vi "MGCC_FntStaMach_Visitualization.vi"() -> ()   [LabVIEW 2016]
uses:
  <vilib>/DNP3/DNP3_Master/Response Type.ctl
  <vilib>/DNP3/DNP3_Master.lvlib
panel:
  in  "S1114-STATUS-CTRL":dbl
  in  "S1011-STATUS-CTRL":dbl
  in  "S0910-STATUS-CTRL":dbl
  in  "S0709-STATUS-CTRL":dbl
  in  "S0708-STATUS-CTRL":dbl
  in  "S0406-STATUS-CTRL":dbl
  in  "S0405-STATUS-CTRL":dbl
  in  "S0307-STATUS-CTRL":dbl
  in  "S0304-STATUS-CTRL":dbl
  in  "S0203-STATUS-CTRL":dbl
  in  "S0102-STATUS-CTRL":dbl
  out "S1114-status":dbl
  out "S1011-status":dbl
  out "S0910-status":dbl
  out "S0709-status":dbl
  out "S0708-status":dbl
  out "S0406-status":dbl
  out "S0405-status":dbl
  out "S0307-status":dbl
  out "S0304-status":dbl
  out "S0203-status":dbl
  out "S0102-status":dbl
  out "f_MGCC_LoadFcst_FcstLoad4":dbl[](array[numeric])
  out "f_MGCC_LoadFcst_FcstLoad2":dbl[](array[numeric])
  out "f_MGCC_LoadFcst_FcstLoad5":dbl[](array[numeric])
  out "f_MGCC_LoadFcst_FcstLoad3":dbl[](array[numeric])
  out "f_MGCC_LoadFcst_FcstLoad1":dbl[](array[numeric])
  out "Comm_MS2_RX_Status_Digital":T1
  out "Comm_MS2_RX_Status_Analog":T1
  out "Comm_MS2_TX_Status_Digital":T1
  out "Comm_MS2_TX_Status_Analog":T1
  out "f_MGCC_EnergyMgmt_ISD_Ppv24":dbl[](array[numeric])
  out "f_MGCC_EnergyMgmt_Pbatt24":dbl[](array[numeric])
  out "Waveform Chart":dbl[](graph)
  out "Model Management":bool
  in  "Ready for STD":bool
  in  "Recon cmd":bool
  in  "BKS cmd":bool
  in  "island cmd":bool
  out "Energy management":bool
  out "BKS":bool
  out "PV Forecasting":bool
  out "Load Forecasting":bool
  out "Communication":bool
  out "PQ Balance":bool
  out "Data Logging":bool
  out "State Estimation":bool
  out "PV Power Output":dbl format="%#_4f"
  out "Angle difference":dbl format="%#_3f"
  out "Angle difference":dbl format="%#_6f"
  in  "Island 2":bool
  out "Sources Power":cluster{"Double":dbl, "Double":dbl}(graph)
  out "Current state":string
  out "10":cluster{dbl[], dbl[]}(graph)
  out "9":cluster{dbl[], dbl[]}(graph)
  out "3":cluster{dbl[], dbl[]}(graph)
  out "4":cluster{dbl[], dbl[]}(graph)
  out "2":cluster{dbl[], dbl[]}(graph)
  out "1":cluster{dbl[], dbl[]}(graph)
  in  "Irradiance":i64(slide) min=0 max=1000 step=500 scale=0.0..1000.0 scale format="%#.0f"
  in  "Island":bool
  in  "RESET":bool
  out "Frequency":dbl(graph)
  out "SW GI2":bool
  out "SW PV1":bool
  out "SW BESS 1":bool
  out "SW3":bool
  out "SW GI1":bool
  out "SW4":bool
  out "SW2":bool
  out "SW1":bool
  out "Loads Power":T2(graph)
  out "Voltage":T3(graph)
  out "BESS Power Output":dbl format="%#_4f"
  # "rad"
  # "rad"
  # "L4"
  # "L6"
  # "L5"
  # "p.u."
  # "+ : Discharging\n-  : Charging"
  # "p.u."
  # "L1"
  # "L3"
  # "L2"
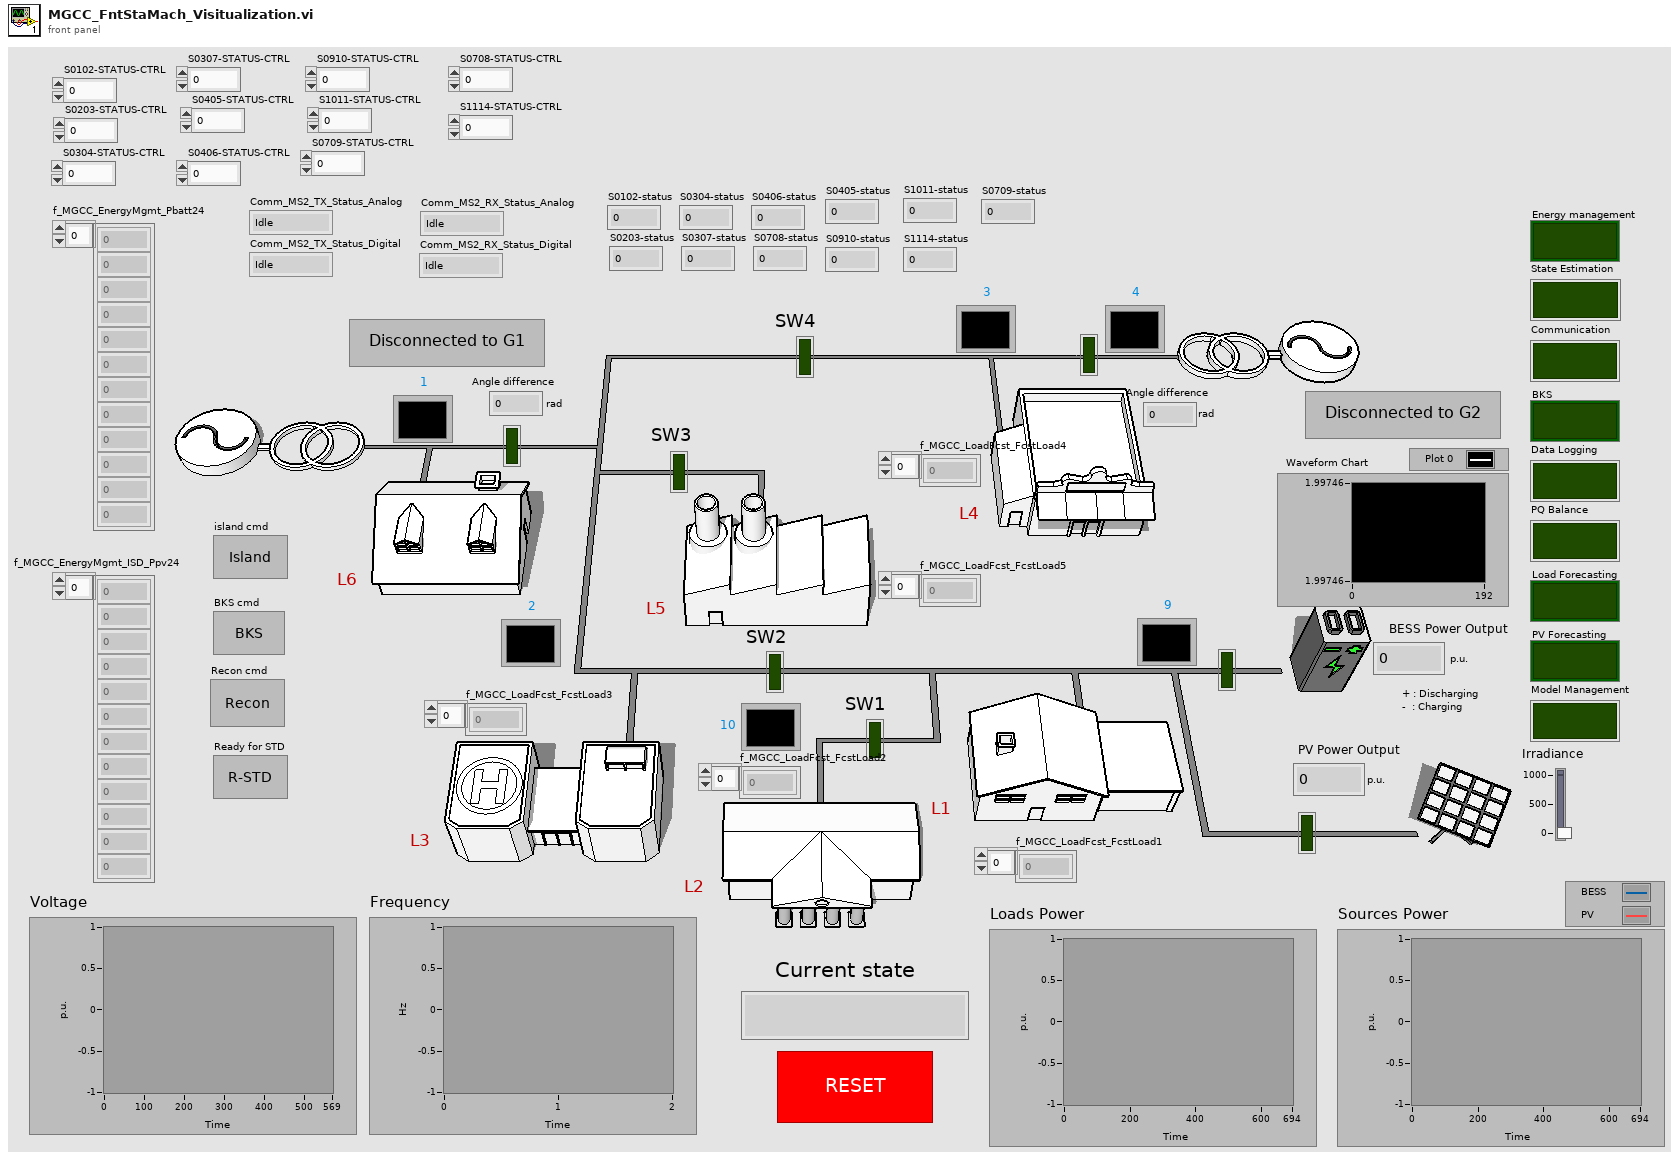
[diagram p1: front panel]
types:
  T1 = typedef "DNP3_Master.lvlib/Response Type.ctl" = enum16{"Idle", "Buffering", "Pending", "Success", "Failure", "Mismatch", "Status Code", "IIN", "Timeout", "Cancel"}
  T2 = cluster{"Double":dbl, "Double":dbl, "Double":dbl, "Double":dbl, "Double":dbl}
  T3 = cluster{"Double":dbl, "Double":dbl, "Double":dbl, "Double":dbl, "Double":dbl, "Double":dbl, "Double":dbl, "Double":dbl, "Double":dbl, "Double":dbl, "Double":dbl, "Double":dbl}
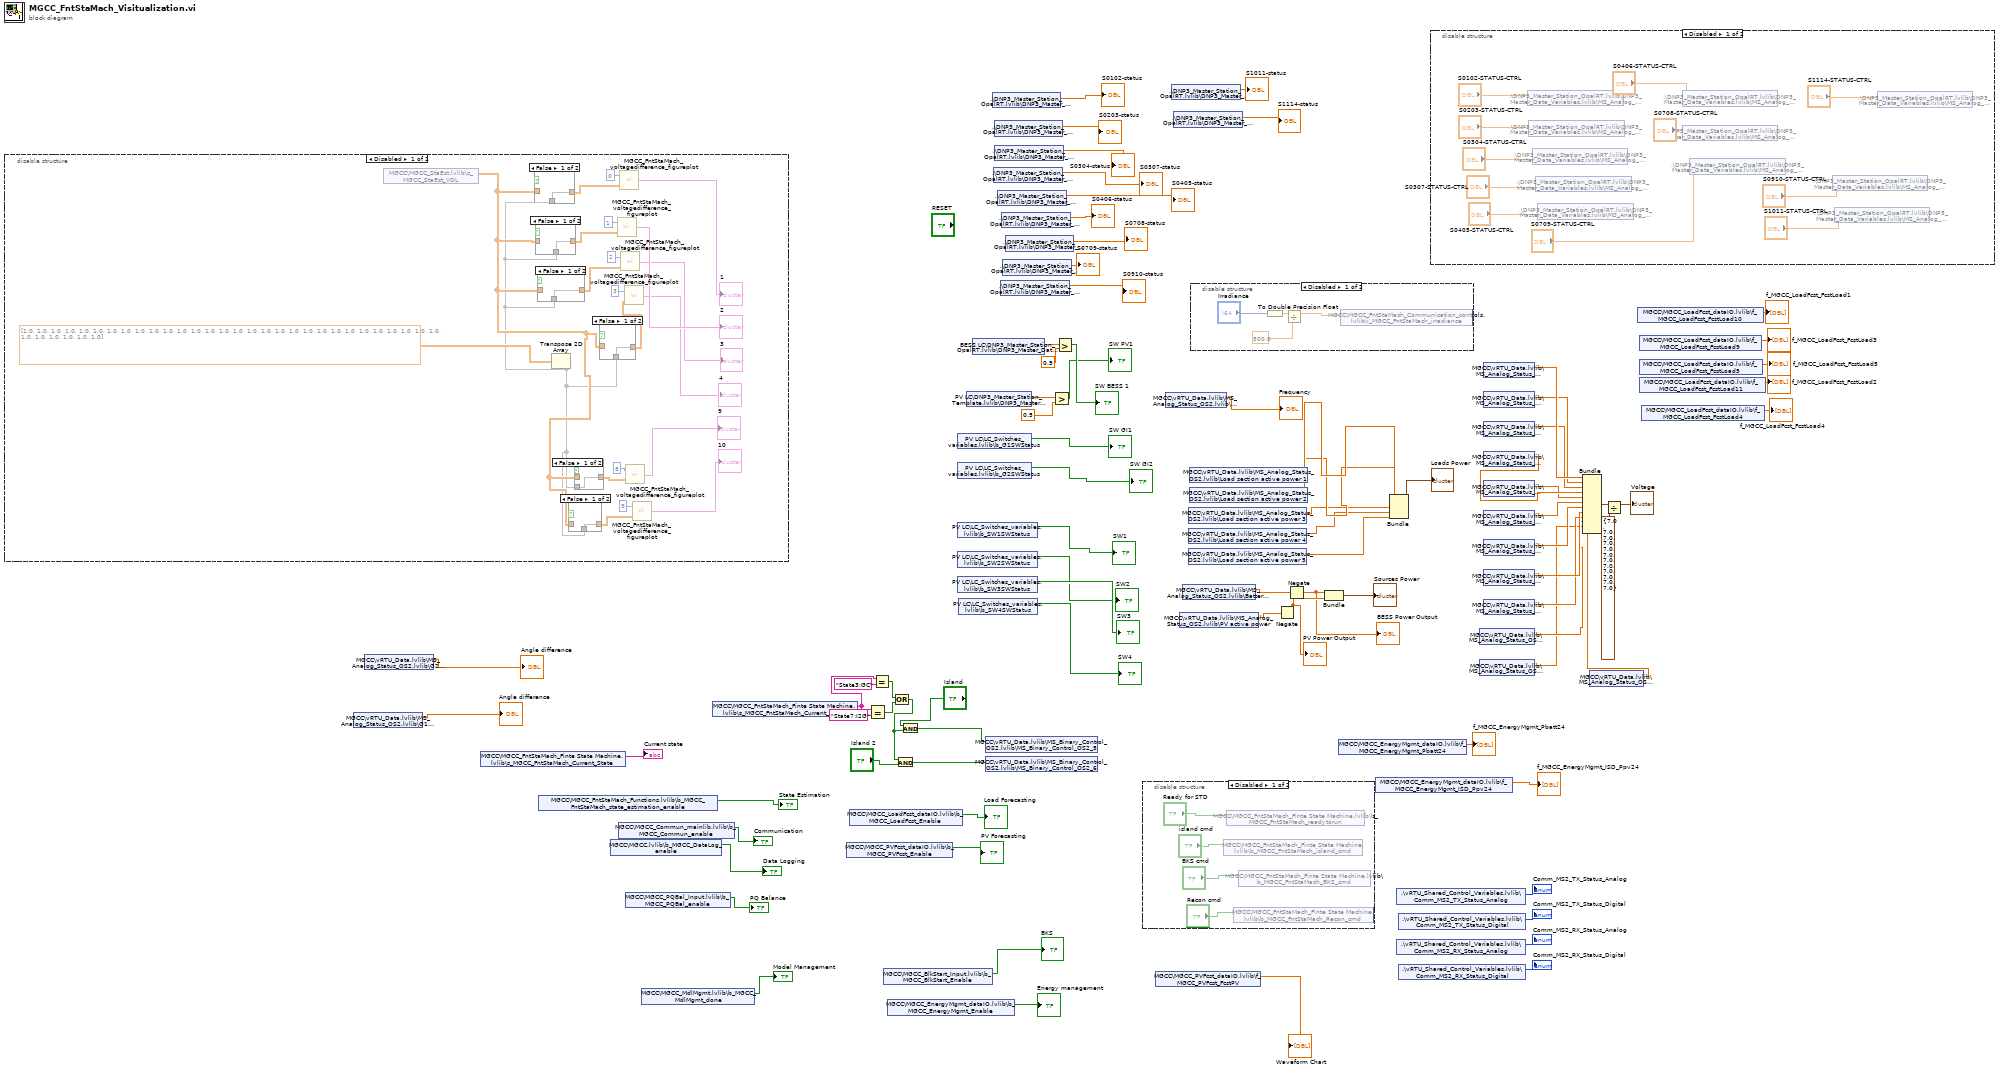
[diagram p0: block diagram]
diagram:
  n1 = disable-structure shown="Disabled" {
    frame Disabled {
      n2 = shared-variable "MGCC\\MGCC_StaEst.lvlib\\c_MGCC_StaEst_VOL"() -> (w87:cdb[][])  [unwired: 1 in, 1 out]
      n3 = Transpose 2D Array(2D array=dbl[][] [[1.0, 1.0, 1.0, 1.0, 1.0, 1.0, 1.0, 1.0, 1.0, 1.0, 1.0, 1.0], [1.0, 1.0, 1.0, 1.0, 1.0, 1.0, 1.0, 1.0, 1.0, 1.0, 1.0, 1.0], [1.0, 1.0, 1.0, 1.0, 1.0, 1.0, 1.0, 1.0, 1.0, 1.0, 1.0, 1.0]] ("lower limit")) -> (transposed array=w85:dbl[][])
      n4 = case shown="False" {
        selector: _ -> [_ _]
        tunnel: w87 -> [_ w113]
        tunnel: [w112 w113] -> w90
        tunnel: w85 -> [w112 _]
        frame False {
        }
        frame True {
        }
      }
      n5 = case shown="False" {
        selector: _ -> [_ _]
        tunnel: w87 -> [_ w111]
        tunnel: [w110 w111] -> w89
        tunnel: w85 -> [w110 _]
        frame False {
        }
        frame True {
        }
      }
      n6 = case shown="False" {
        selector: _ -> [_ _]
        tunnel: w87 -> [_ w109]
        tunnel: [w108 w109] -> w88
        tunnel: w85 -> [w108 _]
        frame False {
        }
        frame True {
        }
      }
      n7 = case shown="False" {
        selector: _ -> [_ _]
        tunnel: w87 -> [_ w115]
        tunnel: [w114 w115] -> w91
        tunnel: w85 -> [w114 _]
        frame False {
        }
        frame True {
        }
      }
      n8 = case shown="False" {
        selector: _ -> [_ _]
        tunnel: w87 -> [_ w117]
        tunnel: [w116 w117] -> w92
        tunnel: w85 -> [w116 _]
        frame False {
        }
        frame True {
        }
      }
      n9 = case shown="False" {
        selector: _ -> [_ _]
        tunnel: w87 -> [_ w107]
        tunnel: [w106 w107] -> w86
        tunnel: w85 -> [w106 _]
        frame False {
        }
        frame True {
        }
      }
      n10 = call "MGCC_FntStaMach_voltagedifference_figureplot.vi"("array"=w89, "index (row)"=1) -> ("output cluster"=→"2":cluster{dbl[], dbl[]})
      n11 = call "MGCC_FntStaMach_voltagedifference_figureplot.vi"("array"=w90, "index (row)"=0) -> ("output cluster"=→"1":cluster{dbl[], dbl[]})
      n12 = call "MGCC_FntStaMach_voltagedifference_figureplot.vi"("array"=w88, "index (row)"=2) -> ("output cluster"=→"3":cluster{dbl[], dbl[]})
      n13 = call "MGCC_FntStaMach_voltagedifference_figureplot.vi"("array"=w86, "index (row)"=3) -> ("output cluster"=→"4":cluster{dbl[], dbl[]})
      n14 = call "MGCC_FntStaMach_voltagedifference_figureplot.vi"("array"=w92, "index (row)"=8) -> ("output cluster"=→"9":cluster{dbl[], dbl[]})
      n15 = call "MGCC_FntStaMach_voltagedifference_figureplot.vi"("array"=w91, "index (row)"=9) -> ("output cluster"=→"10":cluster{dbl[], dbl[]})
    }
    frame Enabled {
    }
  }
  n16 = shared-variable "MGCC\\vRTU_Data.lvlib\\MS_Analog_Status_OS2.lvlib\\G1 angle diff"() -> (→"Angle difference":dbl)  [unwired: 1 in, 1 out]
  n17 = shared-variable "MGCC\\vRTU_Data.lvlib\\MS_Analog_Status_OS2.lvlib\\G2 angle diff"() -> (→"Angle difference":dbl)  [unwired: 1 in, 1 out]
  n18 = shared-variable "MGCC\\MGCC_FntStaMach_Finte State Machine.lvlib\\s_MGCC_FntStaMach_Current_State"() -> (→"Current state":string)  [unwired: 1 in, 1 out]
  n19 = shared-variable "MGCC\\MGCC_FntStaMach_Functions.lvlib\\b_MGCC_FntStaMach_state_estimation_enable"() -> (→"State Estimation":bool)  [unwired: 1 in, 1 out]
  n20 = shared-variable "MGCC\\MGCC.lvlib\\b_MGCC_DataLog_enable"() -> (→"Data Logging":bool)  [unwired: 1 in, 1 out]
  n21 = shared-variable "MGCC\\MGCC_Commun_mainlib.lvlib\\b_MGCC_Commun_enable"() -> (→"Communication":bool)  [unwired: 1 in, 1 out]
  n22 = shared-variable "MGCC\\MGCC_PQBal_Input.lvlib\\b_MGCC_PQBal_enable"() -> (→"PQ Balance":bool)  [unwired: 1 in, 1 out]
  n23 = shared-variable "MGCC\\MGCC_MdlMgmt.lvlib\\b_MGCC_MdlMgmt_done"() -> (→"Model Management":bool)  [unwired: 1 in, 1 out]
  n24 = shared-variable "MGCC\\MGCC_FntStaMach_Finte State Machine.lvlib\\s_MGCC_FntStaMach_Current_State"() -> (w47:string)  [unwired: 1 in, 1 out]
  n25 = shared-variable "MGCC\\MGCC_PVFcst_dataIO.lvlib\\b_MGCC_PVFcst_Enable"() -> (→"PV Forecasting":bool)  [unwired: 1 in, 1 out]
  n26 = shared-variable "MGCC\\MGCC_LoadFcst_dataIO.lvlib\\b_MGCC_LoadFcst_Enable"() -> (→"Load Forecasting":bool)  [unwired: 1 in, 1 out]
  n27 = Equal?(x=w47, y="State7:I2G") -> (x = y?=w46:bool)
  n28 = Equal?(x=w47, y="State3:GC") -> (x = y?=w45:bool)
  n29 = shared-variable "MGCC\\MGCC_BlkStart_Input.lvlib\\b_MGCC_BlkStart_Enable"() -> (→"BKS":bool)  [unwired: 1 in, 1 out]
  n30 = shared-variable "MGCC\\MGCC_EnergyMgmt_dataIO.lvlib\\b_MGCC_EnergyMgmt_Enable"() -> (→"Energy management":bool)  [unwired: 1 in, 1 out]
  n31 = Or(x=w45, y=w46) -> (x .or. y?=w44:bool)
  n32 = And(x=w44, y="Island 2") -> (x .and. y?=w49:bool)
  n33 = And(x="Island", y=w44) -> (x .and. y?=w51:bool)
  n34 = shared-variable "PV LC\\LC_Switches_variables.lvlib\\b_G1SWStatus"() -> (→"SW GI1":bool)  [unwired: 1 in, 1 out]
  n35 = shared-variable "PV LC\\LC_Switches_variables.lvlib\\b_G2SWStatus"() -> (→"SW GI2":bool)  [unwired: 1 in, 1 out]
  n36 = shared-variable "PV LC\\LC_Switches_variables.lvlib\\b_SW1SWStatus"() -> (→"SW1":bool)  [unwired: 1 in, 1 out]
  n37 = shared-variable "PV LC\\LC_Switches_variables.lvlib\\b_SW2SWStatus"() -> (→"SW2":bool)  [unwired: 1 in, 1 out]
  n38 = shared-variable "PV LC\\LC_Switches_variables.lvlib\\b_SW3SWStatus"() -> (→"SW3":bool)  [unwired: 1 in, 1 out]
  n39 = shared-variable "PV LC\\LC_Switches_variables.lvlib\\b_SW4SWStatus"() -> (→"SW4":bool)  [unwired: 1 in, 1 out]
  n40 = shared-variable "PV LC\\DNP3_Master_Station_Template.lvlib\\DNP3_Master_Data_Variables.lvlib\\MS_Analog_Status.lvlib\\PV-STATUS"() -> (w13:dbl)  [unwired: 1 in, 1 out]
  n41 = shared-variable "BESS LC\\DNP3_Master_Station_OpalRT.lvlib\\DNP3_Master_Data_Variables.lvlib\\MS_Analog_Status.lvlib\\BESS-STATUS"() -> (w17:dbl)  [unwired: 1 in, 1 out]
  n42 = shared-variable "MGCC\\vRTU_Data.lvlib\\MS_Binary_Control_OS2.lvlib\\MS_Binary_Control_OS2_5"(w51) -> ()  [unwired: 1 in, 1 out]
  n43 = shared-variable "MGCC\\vRTU_Data.lvlib\\MS_Binary_Control_OS2.lvlib\\MS_Binary_Control_OS2_6"(w49) -> ()  [unwired: 1 in, 1 out]
  n44 = shared-variable ".\\DNP3_Master_Station_OpalRT.lvlib\\DNP3_Master_Data_Variables.lvlib\\MS_Analog_Status.lvlib\\S0102-status"() -> (→"S0102-status":dbl)  [unwired: 1 in, 1 out]
  n45 = shared-variable ".\\DNP3_Master_Station_OpalRT.lvlib\\DNP3_Master_Data_Variables.lvlib\\MS_Analog_Status.lvlib\\S0307-status"() -> (→"S0307-status":dbl)  [unwired: 1 in, 1 out]
  n46 = shared-variable ".\\DNP3_Master_Station_OpalRT.lvlib\\DNP3_Master_Data_Variables.lvlib\\MS_Analog_Status.lvlib\\S0203-status"() -> (→"S0203-status":dbl)  [unwired: 1 in, 1 out]
  n47 = shared-variable ".\\DNP3_Master_Station_OpalRT.lvlib\\DNP3_Master_Data_Variables.lvlib\\MS_Analog_Status.lvlib\\S0304-status"() -> (→"S0304-status":dbl)  [unwired: 1 in, 1 out]
  n48 = shared-variable ".\\DNP3_Master_Station_OpalRT.lvlib\\DNP3_Master_Data_Variables.lvlib\\MS_Analog_Status.lvlib\\S0405-status"() -> (→"S0405-status":dbl)  [unwired: 1 in, 1 out]
  n49 = shared-variable ".\\DNP3_Master_Station_OpalRT.lvlib\\DNP3_Master_Data_Variables.lvlib\\MS_Analog_Status.lvlib\\S0910-status"() -> (→"S0910-status":dbl)  [unwired: 1 in, 1 out]
  n50 = shared-variable ".\\DNP3_Master_Station_OpalRT.lvlib\\DNP3_Master_Data_Variables.lvlib\\MS_Analog_Status.lvlib\\S0406-status"() -> (→"S0406-status":dbl)  [unwired: 1 in, 1 out]
  n51 = shared-variable ".\\DNP3_Master_Station_OpalRT.lvlib\\DNP3_Master_Data_Variables.lvlib\\MS_Analog_Status.lvlib\\S0709-status"() -> (→"S0709-status":dbl)  [unwired: 1 in, 1 out]
  n52 = shared-variable ".\\DNP3_Master_Station_OpalRT.lvlib\\DNP3_Master_Data_Variables.lvlib\\MS_Analog_Status.lvlib\\S0708-status"() -> (→"S0708-status":dbl)  [unwired: 1 in, 1 out]
  n53 = Greater?(x=w13, y=0.5) -> (0:→"SW PV1":bool)
  n54 = Greater?(x=w17, y=0.5) -> (0:→"SW BESS 1":bool)
  n55 = disable-structure shown="Disabled" {
    frame Disabled {
      n56 = shared-variable "MGCC\\MGCC_FntStaMach_Finte State Machine.lvlib\\b_MGCC_FntStaMach_island_cmd"("island cmd") -> ()  [unwired: 1 in, 1 out]
      n57 = shared-variable "MGCC\\MGCC_FntStaMach_Finte State Machine.lvlib\\b_MGCC_FntStaMach_readytorun"("Ready for STD") -> ()  [unwired: 1 in, 1 out]
      n58 = shared-variable "MGCC\\MGCC_FntStaMach_Finte State Machine.lvlib\\b_MGCC_FntStaMach_Recon_cmd"("Recon cmd") -> ()  [unwired: 1 in, 1 out]
      n59 = shared-variable "MGCC\\MGCC_FntStaMach_Finte State Machine.lvlib\\b_MGCC_FntStaMach_BKS_cmd"("BKS cmd") -> ()  [unwired: 1 in, 1 out]
    }
    frame Enabled {
    }
  }
  n60 = shared-variable "MGCC\\MGCC_PVFcst_dataIO.lvlib\\f_MGCC_PVFcst_FcstPV"() -> (→"Waveform Chart":dbl[])  [unwired: 1 in, 1 out]
  n61 = shared-variable "MGCC\\vRTU_Data.lvlib\\MS_Analog_Status_OS2.lvlib\\Frequency"() -> (→"Frequency":dbl)  [unwired: 1 in, 1 out]
  n62 = shared-variable ".\\DNP3_Master_Station_OpalRT.lvlib\\DNP3_Master_Data_Variables.lvlib\\MS_Analog_Status.lvlib\\S1011-status"() -> (→"S1011-status":dbl)  [unwired: 1 in, 1 out]
  n63 = shared-variable ".\\DNP3_Master_Station_OpalRT.lvlib\\DNP3_Master_Data_Variables.lvlib\\MS_Analog_Status.lvlib\\S1114-status"() -> (→"S1114-status":dbl)  [unwired: 1 in, 1 out]
  n64 = shared-variable "MGCC\\vRTU_Data.lvlib\\MS_Analog_Status_OS2.lvlib\\PV active power"() -> (w20:dbl)  [unwired: 1 in, 1 out]
  n65 = shared-variable "MGCC\\vRTU_Data.lvlib\\MS_Analog_Status_OS2.lvlib\\Battery power"() -> (w21:dbl)  [unwired: 1 in, 1 out]
  n66 = shared-variable "MGCC\\vRTU_Data.lvlib\\MS_Analog_Status_OS2.lvlib\\Load section active power 3"() -> (w82:dbl)  [unwired: 1 in, 1 out]
  n67 = shared-variable "MGCC\\vRTU_Data.lvlib\\MS_Analog_Status_OS2.lvlib\\Load section active power 4"() -> (w81:dbl)  [unwired: 1 in, 1 out]
  n68 = shared-variable "MGCC\\vRTU_Data.lvlib\\MS_Analog_Status_OS2.lvlib\\Load section active power 5"() -> (w80:dbl)  [unwired: 1 in, 1 out]
  n69 = shared-variable "MGCC\\vRTU_Data.lvlib\\MS_Analog_Status_OS2.lvlib\\Load section active power 1"() -> (w84:dbl)  [unwired: 1 in, 1 out]
  n70 = shared-variable "MGCC\\vRTU_Data.lvlib\\MS_Analog_Status_OS2.lvlib\\Load section active power 2"() -> (w83:dbl)  [unwired: 1 in, 1 out]
  n71 = disable-structure shown="Disabled" {
    frame Disabled {
      n72 = To Double Precision Float(number="Irradiance") -> (double precision float=w122:dbl)
      n73 = Divide(x=w122, y=500.0) -> (x/y=w124:dbl)
      n74 = shared-variable "MGCC\\MGCC_FntStaMach_Communication_controls.lvlib\\i_MGCC_FntStaMach_irradiance"(w124) -> ()  [unwired: 1 in, 1 out]
    }
    frame Enabled {
    }
  }
  n75 = Negate(x=w20) -> (-x=w57:dbl)
  "PV Power Output" <- w57
  n76 = Negate(x=w21) -> (-x=w56:dbl)
  "BESS Power Output" <- w56
  n77 = Bundle(w56, w57) -> (→"Sources Power":cluster{dbl, dbl})  [unwired: 1 in]
  n78 = shared-variable "MGCC\\MGCC_EnergyMgmt_dataIO.lvlib\\f_MGCC_EnergyMgmt_Pbatt24"() -> (→"f_MGCC_EnergyMgmt_Pbatt24":dbl[])  [unwired: 1 in, 1 out]
  n79 = shared-variable "MGCC\\MGCC_EnergyMgmt_dataIO.lvlib\\f_MGCC_EnergyMgmt_ISD_Ppv24"() -> (→"f_MGCC_EnergyMgmt_ISD_Ppv24":dbl[])  [unwired: 1 in, 1 out]
  n80 = Bundle("Double"=w84, "Double"=w83, "Double"=w82, "Double"=w81, "Double"=w80) -> (→"Loads Power":T2)  [unwired: 1 in]
  n81 = shared-variable ".\\vRTU_Shared_Control_Variables.lvlib\\Comm_MS2_TX_Status_Analog"() -> (→"Comm_MS2_TX_Status_Analog":T1)  [unwired: 1 in, 1 out]
  n82 = shared-variable ".\\vRTU_Shared_Control_Variables.lvlib\\Comm_MS2_RX_Status_Analog"() -> (→"Comm_MS2_RX_Status_Analog":T1)  [unwired: 1 in, 1 out]
  n83 = shared-variable ".\\vRTU_Shared_Control_Variables.lvlib\\Comm_MS2_TX_Status_Digital"() -> (→"Comm_MS2_TX_Status_Digital":T1)  [unwired: 1 in, 1 out]
  n84 = shared-variable ".\\vRTU_Shared_Control_Variables.lvlib\\Comm_MS2_RX_Status_Digital"() -> (→"Comm_MS2_RX_Status_Digital":T1)  [unwired: 1 in, 1 out]
  n85 = disable-structure shown="Disabled" {
    frame Disabled {
      n86 = shared-variable ".\\DNP3_Master_Station_OpalRT.lvlib\\DNP3_Master_Data_Variables.lvlib\\MS_Analog_Control.lvlib\\S0102-STATUS-CTRL"("S0102-STATUS-CTRL") -> ()  [unwired: 1 in, 1 out]
      n87 = shared-variable ".\\DNP3_Master_Station_OpalRT.lvlib\\DNP3_Master_Data_Variables.lvlib\\MS_Analog_Control.lvlib\\S0203-STATUS-CTRL"("S0203-STATUS-CTRL") -> ()  [unwired: 1 in, 1 out]
      n88 = shared-variable ".\\DNP3_Master_Station_OpalRT.lvlib\\DNP3_Master_Data_Variables.lvlib\\MS_Analog_Control.lvlib\\S0304-STATUS-CTRL"("S0304-STATUS-CTRL") -> ()  [unwired: 1 in, 1 out]
      n89 = shared-variable ".\\DNP3_Master_Station_OpalRT.lvlib\\DNP3_Master_Data_Variables.lvlib\\MS_Analog_Control.lvlib\\S0307-STATUS-CTRL"("S0307-STATUS-CTRL") -> ()  [unwired: 1 in, 1 out]
      n90 = shared-variable ".\\DNP3_Master_Station_OpalRT.lvlib\\DNP3_Master_Data_Variables.lvlib\\MS_Analog_Control.lvlib\\S0405-STATUS-CTRL"("S0405-STATUS-CTRL") -> ()  [unwired: 1 in, 1 out]
      n91 = shared-variable ".\\DNP3_Master_Station_OpalRT.lvlib\\DNP3_Master_Data_Variables.lvlib\\MS_Analog_Control.lvlib\\S0406-STATUS-CTRL"("S0406-STATUS-CTRL") -> ()  [unwired: 1 in, 1 out]
      n92 = shared-variable ".\\DNP3_Master_Station_OpalRT.lvlib\\DNP3_Master_Data_Variables.lvlib\\MS_Analog_Control.lvlib\\S0708-STATUS-CTRL"("S0708-STATUS-CTRL") -> ()  [unwired: 1 in, 1 out]
      n93 = shared-variable ".\\DNP3_Master_Station_OpalRT.lvlib\\DNP3_Master_Data_Variables.lvlib\\MS_Analog_Control.lvlib\\S0709-STATUS-CTRL"("S0709-STATUS-CTRL") -> ()  [unwired: 1 in, 1 out]
      n94 = shared-variable ".\\DNP3_Master_Station_OpalRT.lvlib\\DNP3_Master_Data_Variables.lvlib\\MS_Analog_Control.lvlib\\S0910-STATUS-CTRL"("S0910-STATUS-CTRL") -> ()  [unwired: 1 in, 1 out]
      n95 = shared-variable ".\\DNP3_Master_Station_OpalRT.lvlib\\DNP3_Master_Data_Variables.lvlib\\MS_Analog_Control.lvlib\\S1011-STATUS-CTRL"("S1011-STATUS-CTRL") -> ()  [unwired: 1 in, 1 out]
      n96 = shared-variable ".\\DNP3_Master_Station_OpalRT.lvlib\\DNP3_Master_Data_Variables.lvlib\\MS_Analog_Control.lvlib\\S1114-STATUS-CTRL"("S1114-STATUS-CTRL") -> ()  [unwired: 1 in, 1 out]
    }
    frame Enabled {
    }
  }
  n97 = shared-variable "MGCC\\vRTU_Data.lvlib\\MS_Analog_Status_OS2.lvlib\\BusV_10"() -> (w69:dbl)  [unwired: 1 in, 1 out]
  n98 = shared-variable "MGCC\\vRTU_Data.lvlib\\MS_Analog_Status_OS2.lvlib\\BusV_11"() -> (w68:dbl)  [unwired: 1 in, 1 out]
  n99 = shared-variable "MGCC\\vRTU_Data.lvlib\\MS_Analog_Status_OS2.lvlib\\BusV_1"() -> (w78:dbl)  [unwired: 1 in, 1 out]
  n100 = shared-variable "MGCC\\vRTU_Data.lvlib\\MS_Analog_Status_OS2.lvlib\\BusV_2"() -> (w77:dbl)  [unwired: 1 in, 1 out]
  n101 = shared-variable "MGCC\\vRTU_Data.lvlib\\MS_Analog_Status_OS2.lvlib\\BusV_3"() -> (w76:dbl)  [unwired: 1 in, 1 out]
  n102 = shared-variable "MGCC\\vRTU_Data.lvlib\\MS_Analog_Status_OS2.lvlib\\BusV_4"() -> (w75:dbl)  [unwired: 1 in, 1 out]
  n103 = shared-variable "MGCC\\vRTU_Data.lvlib\\MS_Analog_Status_OS2.lvlib\\BusV_5"() -> (w74:dbl)  [unwired: 1 in, 1 out]
  n104 = shared-variable "MGCC\\vRTU_Data.lvlib\\MS_Analog_Status_OS2.lvlib\\BusV_6"() -> (w73:dbl)  [unwired: 1 in, 1 out]
  n105 = shared-variable "MGCC\\vRTU_Data.lvlib\\MS_Analog_Status_OS2.lvlib\\BusV_7"() -> (w72:dbl)  [unwired: 1 in, 1 out]
  n106 = shared-variable "MGCC\\vRTU_Data.lvlib\\MS_Analog_Status_OS2.lvlib\\BusV_8"() -> (w71:dbl)  [unwired: 1 in, 1 out]
  n107 = shared-variable "MGCC\\vRTU_Data.lvlib\\MS_Analog_Status_OS2.lvlib\\BusV_9"() -> (w70:dbl)  [unwired: 1 in, 1 out]
  n108 = shared-variable "MGCC\\vRTU_Data.lvlib\\MS_Analog_Status_OS2.lvlib\\BusV_12"() -> (w65:dbl)  [unwired: 1 in, 1 out]
  n109 = Bundle("Double"=w78, "Double"=w77, "Double"=w76, "Double"=w75, "Double"=w74, "Double"=w73, "Double"=w72, "Double"=w71, "Double"=w70, "Double"=w69, "Double"=w68, "Double"=w65) -> (w67:T3)  [unwired: 1 in]
  n110 = Divide(x=w67, y=T3 {"Double"=7.0, "Double"=7.0, "Double"=7.0, "Double"=7.0, "Double"=7.0, "Double"=7.0, "Double"=7.0, "Double"=7.0, "Double"=7.0, "Double"=7.0, "Double"=7.0, "Double"=7.0}) -> (x/y=→"Voltage":T3)
  n111 = shared-variable "MGCC\\MGCC_LoadFcst_dataIO.lvlib\\f_MGCC_LoadFcst_FcstLoad10"() -> (→"f_MGCC_LoadFcst_FcstLoad1":dbl[])  [unwired: 1 in, 1 out]
  n112 = shared-variable "MGCC\\MGCC_LoadFcst_dataIO.lvlib\\f_MGCC_LoadFcst_FcstLoad9"() -> (→"f_MGCC_LoadFcst_FcstLoad3":dbl[])  [unwired: 1 in, 1 out]
  n113 = shared-variable "MGCC\\MGCC_LoadFcst_dataIO.lvlib\\f_MGCC_LoadFcst_FcstLoad11"() -> (→"f_MGCC_LoadFcst_FcstLoad2":dbl[])  [unwired: 1 in, 1 out]
  n114 = shared-variable "MGCC\\MGCC_LoadFcst_dataIO.lvlib\\f_MGCC_LoadFcst_FcstLoad5"() -> (→"f_MGCC_LoadFcst_FcstLoad5":dbl[])  [unwired: 1 in, 1 out]
  n115 = shared-variable "MGCC\\MGCC_LoadFcst_dataIO.lvlib\\f_MGCC_LoadFcst_FcstLoad4"() -> (→"f_MGCC_LoadFcst_FcstLoad4":dbl[])  [unwired: 1 in, 1 out]
